vi "LEP_RV_WriteRuntimeValuesIntoXML.vi"(1 "Execution time":string, 2 "Stack high water mark":string, 3 "Heap high water mark":string) -> (0 "error out":errorcluster)   [LabVIEW 2011]
uses:
  LEP_RV_LaunchGlobals.vi
  <vilib>/xml/Load XML File.vi
  <vilib>/xml/Close Reference(Node).vi
  resource/objmgr/DOMUserDefRef.rc
  <vilib>/xml/NI_XML.lvlib
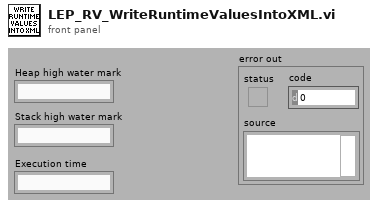
[diagram p1: front panel]
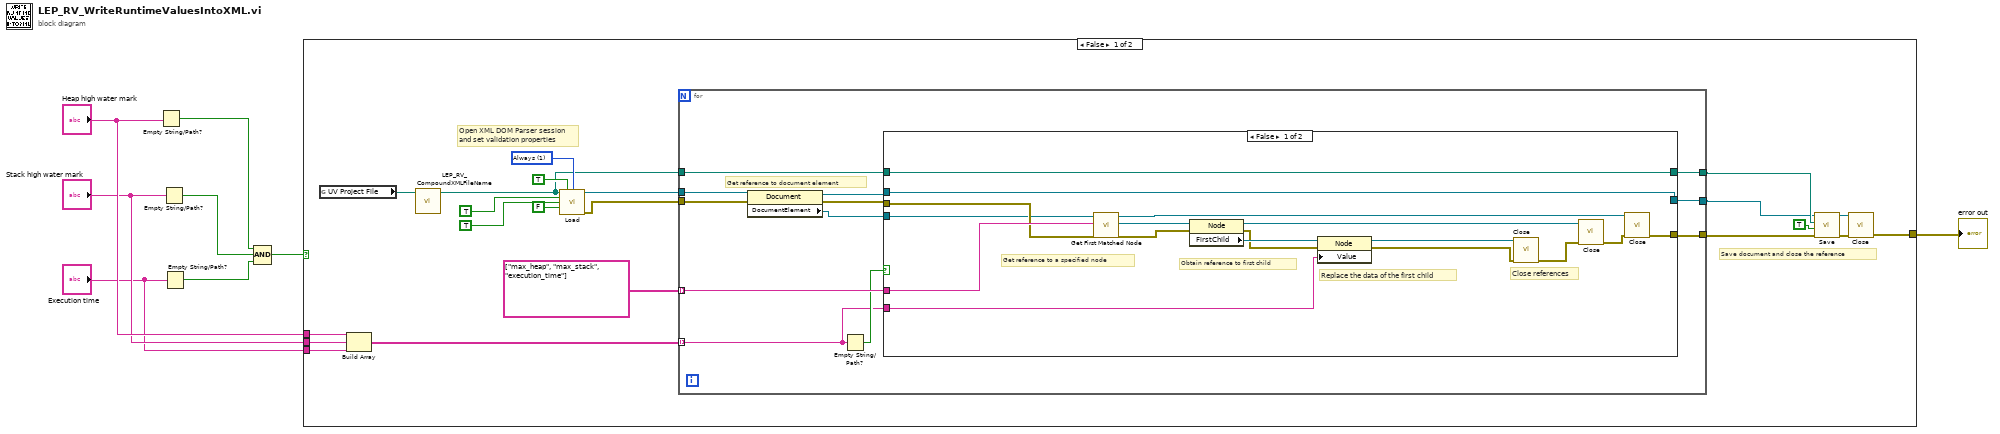
[diagram p0: block diagram]
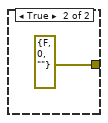
[diagram p3: hidden frame]
diagram:
  n1 = Empty String/Path?(string/path="Heap high water mark") -> (empty?=w8:bool)
  n2 = Empty String/Path?(string/path="Stack high water mark") -> (empty?=w7:bool)
  n3 = Empty String/Path?(string/path="Execution time") -> (empty?=w6:bool)
  n4 = Compound Arithmetic op=AND(w8, w7, w6) -> (w5:bool)
  n5 = case shown="False" w5 {
    tunnel: "Heap high water mark" -> [w27 _]
    tunnel: "Stack high water mark" -> [w29 _]
    tunnel: "Execution time" -> [w28 _]
    tunnel: [w9 errorcluster {"status"=FALSE, "code"=0, "source"=""} ("error out")] -> w1
    frame False {
      w22 = 1 items=["Never", "Always", "Auto"] ("Validate On Load")
      # "Save document and close the reference"
      # "Open XML DOM Parser session\nand set validation properties"
      n6 = global read "LEP_RV_LaunchGlobals.vi" "UV Project File"() -> (w26:path)
      n7 = Build Array(w27, w29, w28) -> (w19:string[])
      n8 = call "LEP_RV_CompoundXMLFileName.vi"("Project file path"=w26) -> ("Path for XML generated file"=w11:path)  [unwired: 10 in]
      n9 = call-poly <vilib>:"Load.vi"("path to XML document"=w11, "preserve whitespace (True)"=TRUE ("Preserve Whitespace"), "validate on load (Auto)"=w22, "process namespaces (False)"=TRUE ("Do Namespaces"), "process schema (False)"=TRUE ("Do Schema"), "load external DTD (True)"=FALSE ("Load External DTD")) -> ("DOM document out"=w12:refnum<k20>, "error out"=w10:errorcluster)  [unwired: 1 in, 7 out]
      n10 = for {
        tunnel: w12 -> [w34]
        tunnel: string[] ["max_heap", "max_stack", "execution_time"] ("delimiters (\\s,\\t,\\r,\\n)") -> [w40] mode=indexing
        tunnel: w19 -> [w38] mode=indexing
        tunnel: w11 -> [w41]
        tunnel: [w37] -> w15
        tunnel: [w36] -> w14
        tunnel: [w35] -> w13
        tunnel: w10 -> [w30]
        # "Get reference to document element"
        n11 = property class="Document"(reference=w34, error in=w30) -> (reference out=w33:refnum<k20>, error out=w31:errorcluster, "DocumentElement"=w32:refnum<k20>)
        n12 = Empty String/Path?(string/path=w38) -> (empty?=w39:bool)
        n13 = case shown="False" w39 {
          tunnel: [w54 w61] -> w35
          tunnel: w33 -> [w50 w59]
          tunnel: w41 -> [w56 w60]
          tunnel: w40 -> [w58 _]
          tunnel: w31 -> [w57 w61]
          tunnel: w38 -> [w47 _]
          tunnel: [w56 w60] -> w37
          tunnel: [w50 w59] -> w36
          tunnel: w32 -> [w53 _]
          frame False {
            # "Get reference to a specified node"
            # "Replace the data of the first child"
            # "Obtain reference to first child"
            # "Close references"
            n14 = call <vilib>:"Get First Matched Node.vi"("error in (no error)"=w57, "XPath expression"=w58, "node in"=w53) -> ("error out"=w51:errorcluster, "node result"=w49:refnum<k20>, "node out"=w48:refnum<k20>)  [unwired: 6 in]
            n15 = property class="Node"(reference=w49, error in=w51) -> (reference out=w52:refnum<k20>, error out=w45:errorcluster, "FirstChild"=w46:refnum<k20>)
            n16 = property class="Node"(reference=w46, error in=w45, "Value"=w47) -> (reference out=w44:refnum<k20>, error out=w42:errorcluster)
            n17 = call-poly <vilib>:"Close.vi"("error in (no error)"=w42, "node"=w44) -> ("error out"=w43:errorcluster)  [unwired: 7 out]
            n18 = call-poly <vilib>:"Close.vi"("error in (no error)"=w43, "node"=w52) -> ("error out"=w55:errorcluster)  [unwired: 7 out]
            n19 = call-poly <vilib>:"Close.vi"("error in (no error)"=w55, "node"=w48) -> ("error out"=w54:errorcluster)  [unwired: 7 out]
          }
          frame True {
          }
        }
      }
      n20 = call <vilib>:"Save.vi"("error in (no error)"=w13, "overwrite file (True)"=TRUE ("Overwrite File (T)"), "XML file path"=w15, "DOM document in"=w14) -> ("error out"=w17:errorcluster, "DOM document out"=w16:refnum<k20>)  [unwired: 6 out]
      n21 = call-poly <vilib>:"Close.vi"("error in (no error)"=w17, "node"=w16) -> ("error out"=w9:errorcluster)  [unwired: 7 out]
    }
    frame True {
    }
  }
  "error out" <- w1
